vi "Queue_Driver.vi"(0 "State_In":string, 2 "Queue_Name_In":string, 5 "N_State_In":string[](array[string]), 7 "Time_Out_In_ms (10)":i32=10, 9 "Max_Queue_Size_In":i32=-1, 11 "Error_In":errorcluster, 13 "Queue_Operation_Select":T1=enum."Flush") -> (4 "State_Out":string, 15 "Error_Out":errorcluster)   [LabVIEW 2023]
doc: "Used to send the states data from one loop to another."
uses:
  Controls/Queue_Operation_Select.ctl
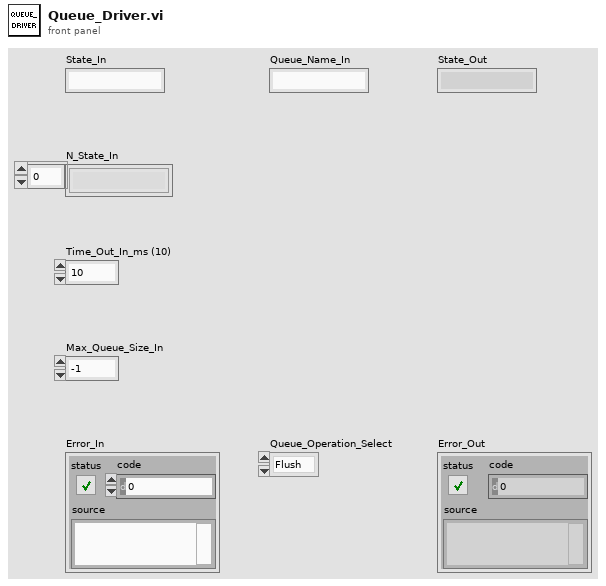
[diagram p1: front panel]
types:
  T1 = typedef "Queue_Operation_Select.ctl" = enum16{"Obtain_Queue", "Enqueue", "Enqueue_N", "Enqueue_at_End", "Dequeue", "Flush", "Release_Queue"}
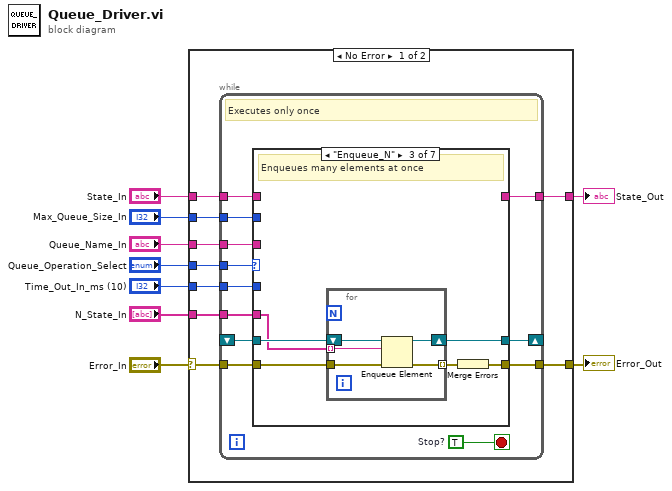
[diagram p0: block diagram]
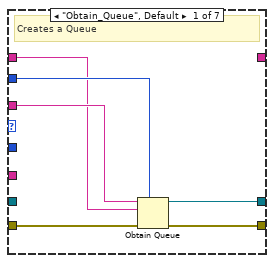
[diagram p2: hidden frame]
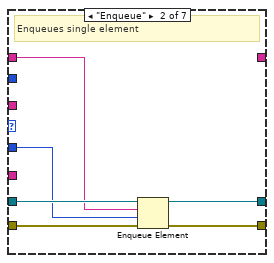
[diagram p3: hidden frame]
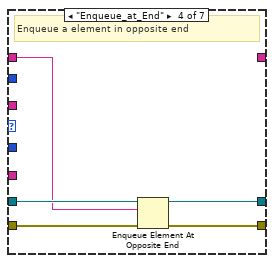
[diagram p4: hidden frame]
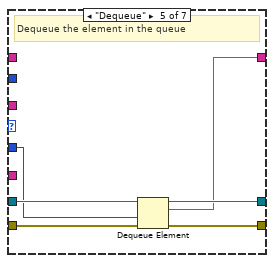
[diagram p5: hidden frame]
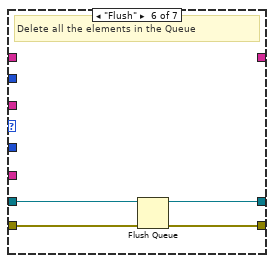
[diagram p6: hidden frame]
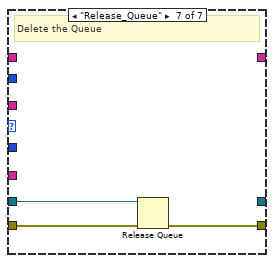
[diagram p7: hidden frame]
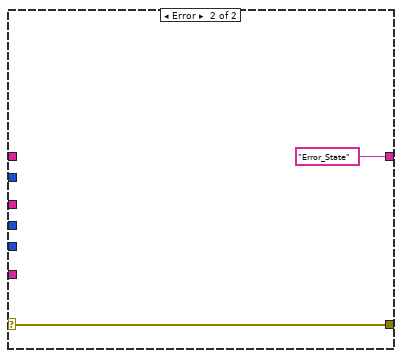
[diagram p8: hidden frame]
diagram:
  n1 = case shown="No Error" "Error_In" {
    selector: "Error_In" -> [w10 w73]
    tunnel: "N_State_In" -> [w18 _]
    tunnel: "Time_Out_In_ms (10)" -> [w17 _]
    tunnel: "Queue_Operation_Select" -> [w16 _]
    tunnel: "Queue_Name_In" -> [w15 _]
    tunnel: "Max_Queue_Size_In" -> [w14 _]
    tunnel: "State_In" -> [w13 _]
    tunnel: [w12 "Error_State" ("State?")] -> w3
    tunnel: [w11 w73] -> w2
    frame No Error {
      n2 = while {
        tunnel: w10 -> [w30]
        tunnel: w18 -> [w29]
        tunnel: w17 -> [w28]
        tunnel: w16 -> [w27]
        tunnel: w15 -> [w26]
        tunnel: w14 -> [w25]
        tunnel: w13 -> [w24]
        tunnel: [w23] -> w12
        tunnel: [w22] -> w11
        shift-right: [w20] -> _
        shift-left: _ -> [w21]
        stop <- w19 stop-if-true
        w19 = TRUE  # Stop?
        # "Executes only once"
        n3 = case shown="\"Enqueue_N\"" w27 {
          tunnel: w30 -> [w36 w42 w44 w57 w63 w67 w70]
          tunnel: w26 -> [w34 _ _ _ _ _ _]
          tunnel: w25 -> [w33 _ _ _ _ _ _]
          tunnel: [w31 w38 w47 w56 w62 w66 _] -> w20
          tunnel: [w35 w41 w43 w55 w60 w65 w69] -> w22
          tunnel: w21 -> [_ w40 w48 w58 w64 w68 w71]
          tunnel: w24 -> [w32 w39 _ w54 _ _ _]
          tunnel: w28 -> [_ w37 _ _ w59 _ _]
          tunnel: [_ _ _ _ w61 _ _] -> w23
          tunnel: w29 -> [_ _ w45 _ _ _ _]
          frame "Obtain_Queue", Default {
            # "Creates a Queue"
            n4 = Obtain Queue(max queue size (-1, unlimited)=w33, name (unnamed)=w34, element data type=w32, error in (no error)=w36) -> (queue out=w31:refnum<queue>, error out=w35:errorcluster)  [unwired: 1 in, 1 out]
          }
          frame "Enqueue" {
            # "Enqueues single element"
            n5 = Enqueue Element(queue=w40, element=w39, timeout in ms (-1)=w37, error in (no error)=w42) -> (queue out=w38:refnum<queue>, error out=w41:errorcluster)  [unwired: 1 out]
          }
          frame "Enqueue_N" {
            # "Enqueues many elements at once"
            n6 = for {
              tunnel: w45 -> [w49] mode=indexing
              tunnel: w44 -> [w52]
              tunnel: [w50] -> w46 mode=indexing
              shift-right: [w51] -> w47
              shift-left: w48 -> [w53]
              n7 = Enqueue Element(queue=w53, element=w49, error in (no error)=w52) -> (queue out=w51:refnum<queue>, error out=w50:errorcluster)  [unwired: 1 in, 1 out]
            }
            n8 = Merge Errors(w46) -> (w43:errorcluster)
          }
          frame "Enqueue_at_End" {
            # "Enqueue a element in opposite end"
            n9 = Enqueue Element At Opposite End(queue=w58, element=w54, error in (no error)=w57) -> (queue out=w56:refnum<queue>, error out=w55:errorcluster)  [unwired: 1 in, 1 out]
          }
          frame "Dequeue" {
            # "Dequeue the element in the queue"
            n10 = Dequeue Element(queue=w64, timeout in ms (-1)=w59, error in (no error)=w63) -> (queue out=w62:refnum<queue>, element=w61:string, error out=w60:errorcluster)  [unwired: 1 out]
          }
          frame "Flush" {
            # "Delete all the elements in the Queue"
            n11 = Flush Queue(queue=w68, error in (no error)=w67) -> (queue out=w66:refnum<queue>, error out=w65:errorcluster)  [unwired: 1 out]
          }
          frame "Release_Queue" {
            # "Delete the Queue"
            n12 = Release Queue(queue=w71, error in (no error)=w70) -> (error out=w69:errorcluster)  [unwired: 1 in, 2 out]
          }
        }
      }
    }
    frame Error {
    }
  }
  "Error_Out" <- w2
  "State_Out" <- w3
